vi "Init Events.vi"(8 "error in (no error)":errorcluster, 11 "ButtonControlEditorPanel in":refnum<class "ButtonControlEditorPanel.lvclass">) -> (0 "error out":errorcluster, 3 "ButtonControlEditorPanel out":refnum<class "ButtonControlEditorPanel.lvclass">)   [LabVIEW 2020]
uses:
  ButtonControlEditorPanel.lvclass
  ButtonControlEditorPanel.lvclass/ButtonControlEditorPanel.ctl
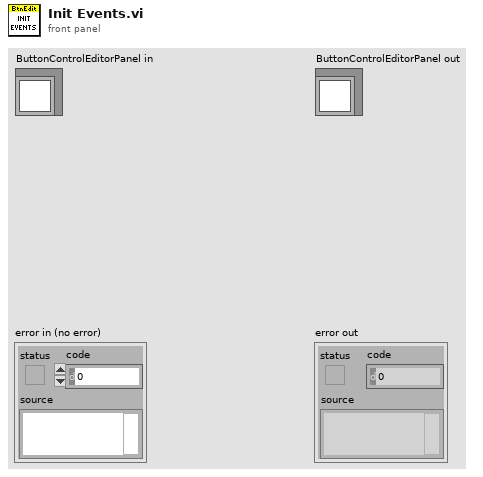
[diagram p1: front panel]
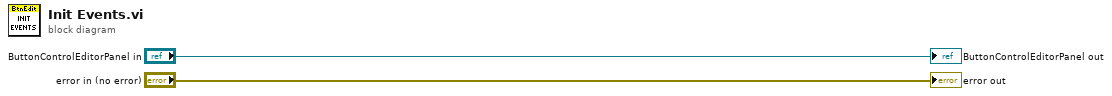
[diagram p0: block diagram]
diagram:
  "error out" <- "error in (no error)"
  "ButtonControlEditorPanel out" <- "ButtonControlEditorPanel in"
